vi "Connect to DB.vi"(8 "error in":errorcluster, 11 "Data Cluster in":T1) -> (0 "error out":errorcluster, 3 "Data Cluster out":T1)   [LabVIEW 2014, in "DB_CONNECTOR.lvlib"]
doc: "Establish a connection to the database."
uses:
  DB_CONNECTOR.lvlib
  Module Data--cluster.ctl
  DB-Interface/DB-Interface.lvclass
  DB-Interface/DB-MySQL/Network Config.ctl
  DB-Interface/DB-MySQL/DB-MySQL.lvclass
  DB-Interface/DB-ADO/DB-ADO.lvclass
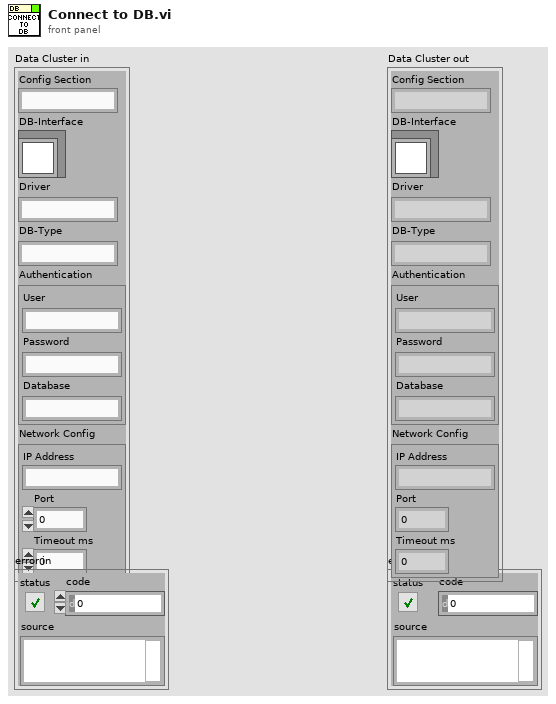
[diagram p1: front panel]
types:
  T1 = typedef "DB_CONNECTOR.lvlib/Module Data--cluster.ctl" = cluster{"Config Section":string, "DB-Interface":refnum<class "DB-Interface.lvclass">, "Driver":string, "DB-Type":string, "Authentication":cluster{"User":string, "Password":string, "Database":string}, "Network Config":T2}
  T2 = typedef "hse-db.lvlib/DB-MySQL.lvclass/Network Config.ctl" = cluster{"IP Address":string, "Port":u16, "Timeout ms":i32}
  T3 = cluster{"User":string, "Password":string, "Database":string}
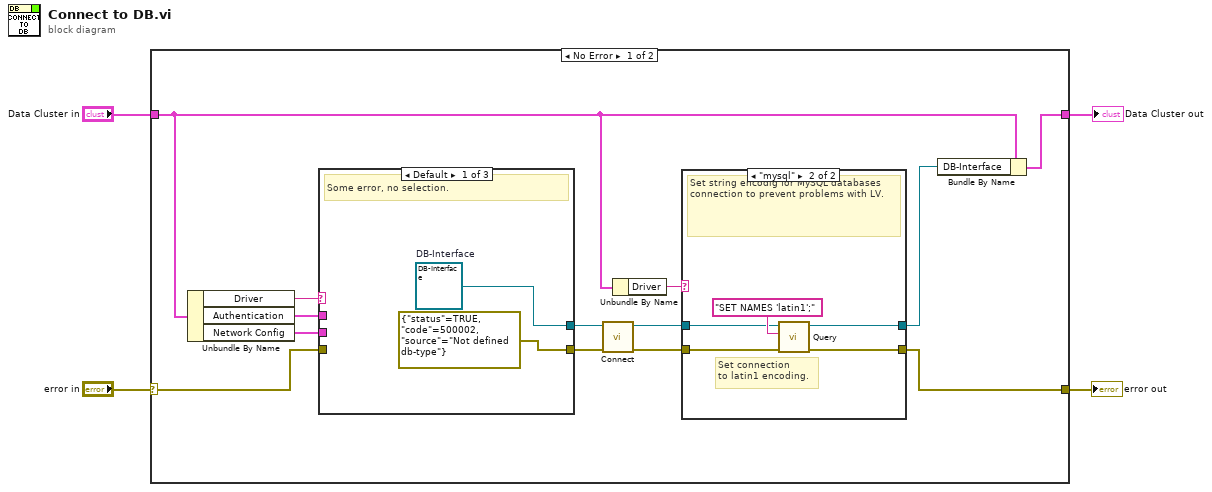
[diagram p0: block diagram]
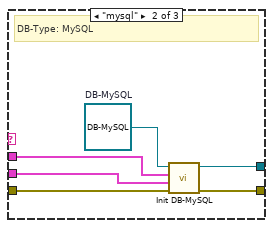
[diagram p3: hidden frame]
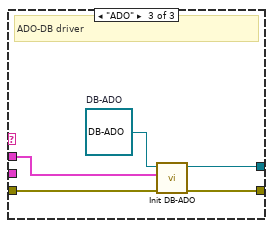
[diagram p4: hidden frame]
diagram:
  n1 = case shown="No Error" "error in" {
    selector: "error in" -> [w7 w39]
    tunnel: [w17 w39] -> w4
    tunnel: [w15 w38] -> w3
    tunnel: "Data Cluster in" -> [w6 w38]
    frame No Error {
      n2 = Unbundle By Name(w6) -> ("Driver"=w8:string, "Authentication"=w9:T3, "Network Config"=w10:T2)
      n3 = case shown="Default" w8 {
        tunnel: [w25 w28 w35] -> w12
        tunnel: w7 -> [_ w32 w37]
        tunnel: w9 -> [_ w30 w34]
        tunnel: w10 -> [_ w31 _]
        tunnel: [errorcluster {"status"=TRUE, "code"=500002, "source"="Not defined db-type"} ("error out") w29 w36] -> w11
        frame Default {
          w25 = refnum<class "DB-Interface.lvclass"> refnum  # DB-Interface
          # "Some error, no selection."
        }
        frame "mysql" {
          w27 = refnum<class "DB-MySQL.lvclass"> refnum  # DB-MySQL
          # "DB-Type: MySQL"
          n4 = call-dynamic "Init DB-MySQL.vi"("error in"=w32, "Network Config"=w31, "Authentication"=w30, "DB-MySQL in"=w27) -> ("error out"=w29:errorcluster, "DB-MySQL out"=w28:refnum<class "DB-MySQL.lvclass">)  [unwired: 6 in]
        }
        frame "ADO" {
          w33 = refnum<class "DB-ADO.lvclass"> refnum  # DB-ADO
          # "ADO-DB driver"
          n5 = call-dynamic "Init DB-ADO.vi"("error in"=w37, "Authentication"=w34, "DB-ADO in"=w33) -> ("error out"=w36:errorcluster, "DB-ADO out"=w35:refnum<class "DB-ADO.lvclass">)  [unwired: 7 in]
        }
      }
      n6 = call-dynamic "Connect.vi"("error in"=w11, "DB-Engine in"=w12) -> ("error out"=w13:errorcluster, "DB-Engine out"=w14:refnum<class "DB-Interface.lvclass">)  [unwired: 8 in]
      n7 = Unbundle By Name(w6) -> ("Driver"=w5:string)
      n8 = case shown="\"mysql\"" w5 {
        tunnel: [w18 w24] -> w17
        tunnel: [w19 w23] -> w16
        tunnel: w14 -> [w19 w21]
        tunnel: w13 -> [w18 w20]
        frame Default {
          # "All other."
        }
        frame "mysql" {
          # "Set connection\nto latin1 encoding."
          # "Set string encodig for MySQL databases connection to prevent problems with LV."
          n9 = call-dynamic "Query.vi"("error in"=w20, "Query"="SET NAMES 'latin1';", "DB-Engine in"=w21) -> ("error out"=w24:errorcluster, "DB-Engine out"=w23:refnum<class "DB-Interface.lvclass">)  [unwired: 4 in, 3 out]
        }
      }
      n10 = Bundle By Name(cluster=w6, "DB-Interface"=w16) -> (w15:T1)
    }
    frame Error {
    }
  }
  "error out" <- w4
  "Data Cluster out" <- w3
